vi "Event handler-Start Stop.vi"(9 "Next State":T1, 11 "UI queue":refnum<queue>) -> (0 "error out":errorcluster, 3 "Queue out":refnum<queue>)   [LabVIEW 2017]
uses:
  Queue/Message Queue/Typedefs/Message Cluster.ctl
  Typedefs/Top level VI states.ctl
  Typedefs/Set Main VI cursor.ctl
  Typedefs/Imaging Protocols enum.ctl
  Typedefs/Start-Stop Enum.ctl
  Global Variables/General Globals.vi
panel:
  # "<---Funct acq fix"
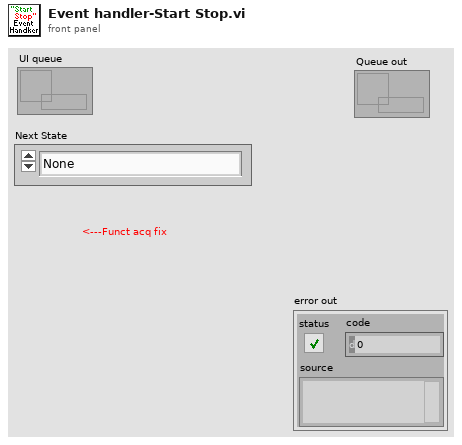
[diagram p1: front panel]
types:
  T1 = typedef "Top level VI states.ctl" = enum16{"None", "Initialise UI", "<STACK PROTOCOL STATES>", "AOL Zstack-START", "AOL Zstack-STOP", "Motor Zstack-START", "Motor Zstack-STOP", "<ACQUISITION PROTOCOL STATES> ", "Functional Acquisition-START", "Functional Acquisition-STOP", "Single Plane Acquisition-START", "Single Plane Acquisition-STOP", "Volume Acquisition-START", "Volume Acquisition-STOP", "<LIVE IMAGING PROTOCOL STATES>", "Live Imaging-START", "Live Imaging-STOP", "Live Plane Imaging-START", "Live Plane Imaging-STOP", "Live Volume Imaging-START", "Live Volume Imaging-STOP", "<MOVEMENT CORRECTION PROTOCOL STATES>", "EXIT"}
  T2 = typedef "Set Main VI cursor.ctl" = enum16{"Release busy cursor", "Set busy cursor"}
  T3 = typedef "Imaging Protocols enum.ctl" = enum16{"AOL Z-Stack", "Motor Z Stack", "Functional Acquisition", "Single Plane Acquisition", "Volume Acquisition", "Live Imaging", "Live Plane Imaging", "Live Volume Imaging"}
  T4 = typedef "Start-Stop Enum.ctl" = enum16{"START", "STOP"}
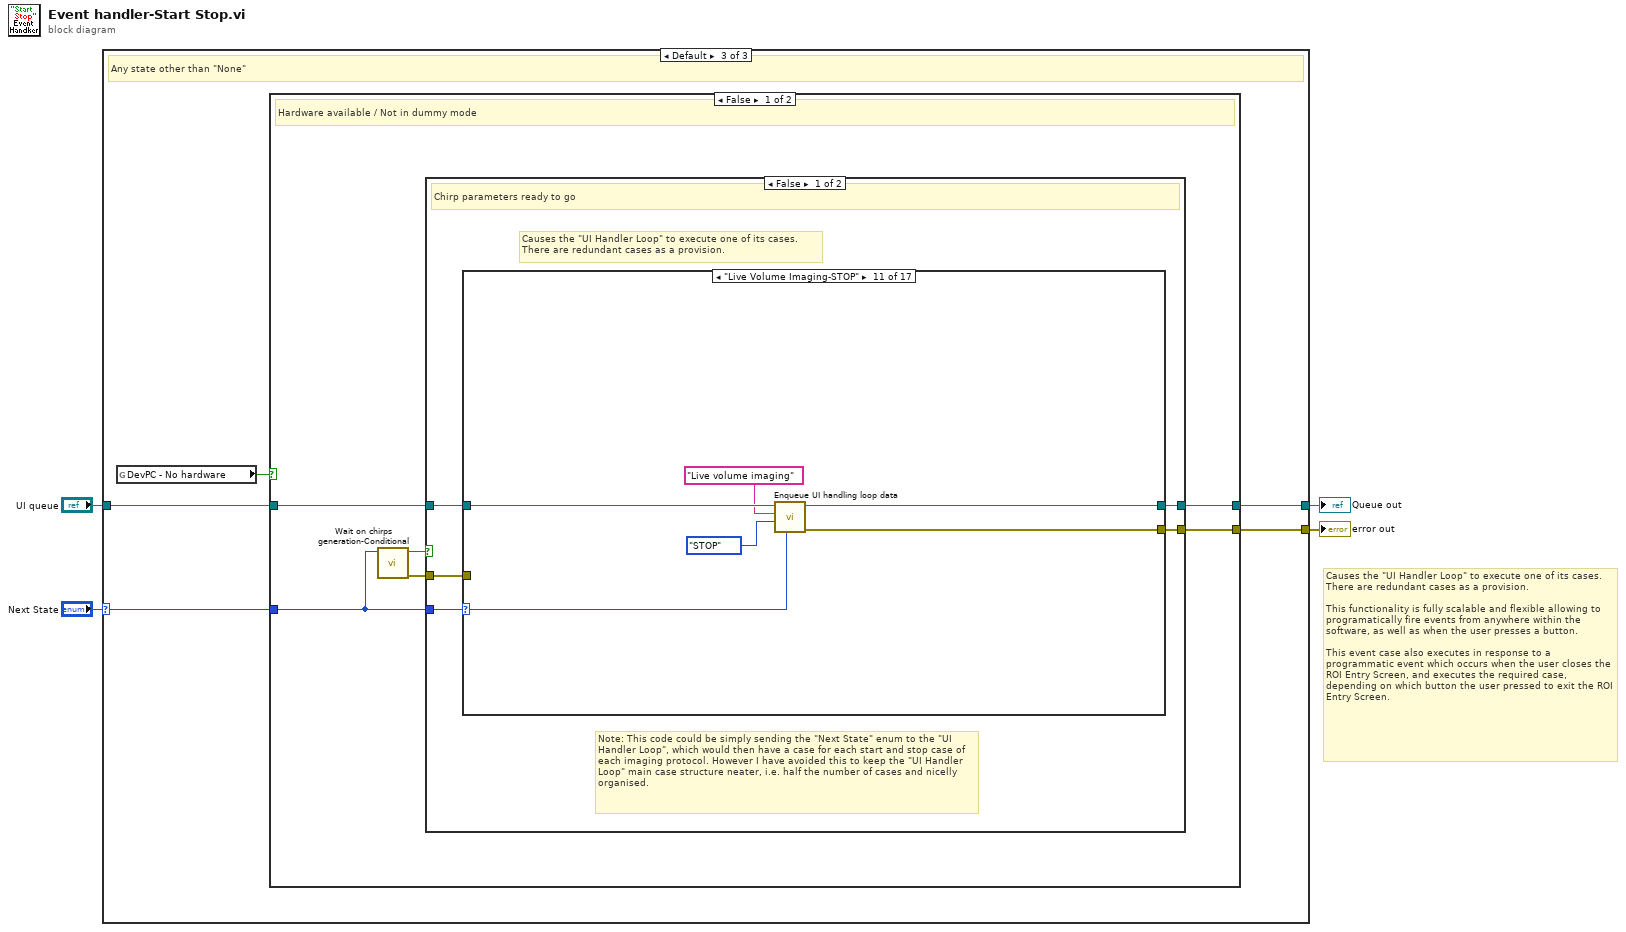
[diagram p0: block diagram]
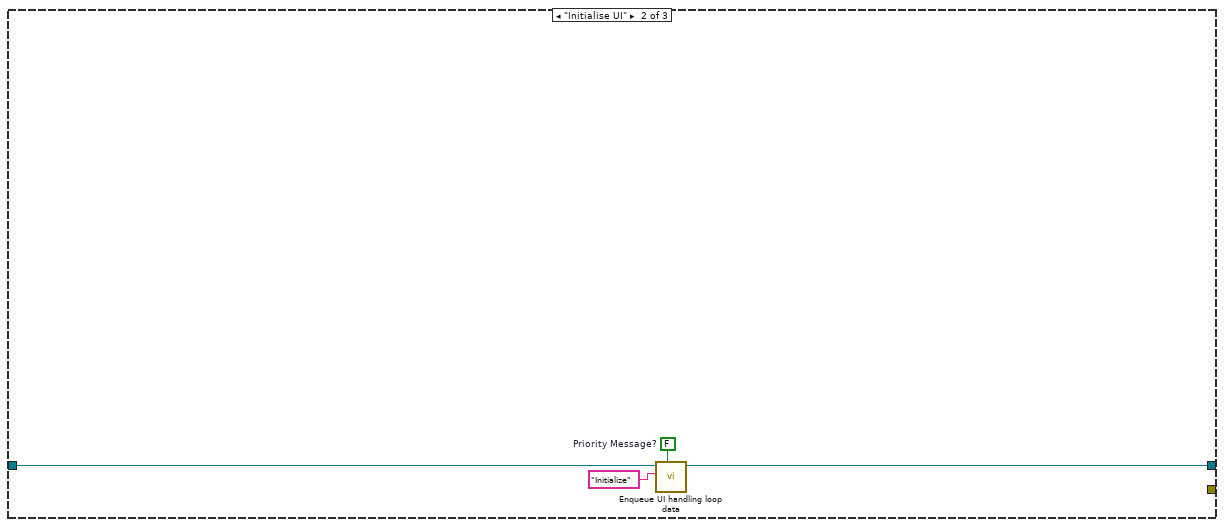
[diagram p3: hidden frame]
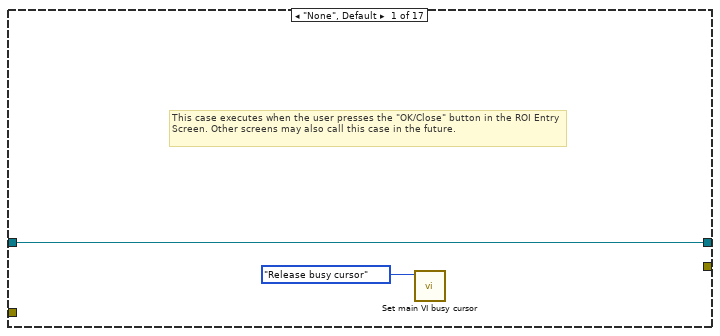
[diagram p4: hidden frame]
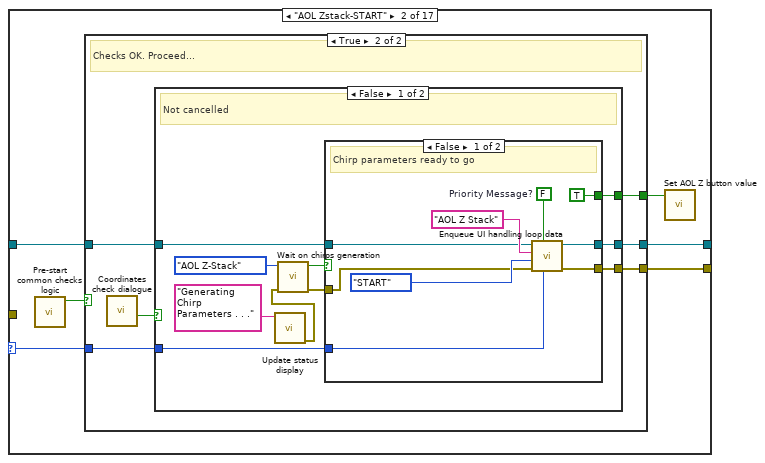
[diagram p5: hidden frame]
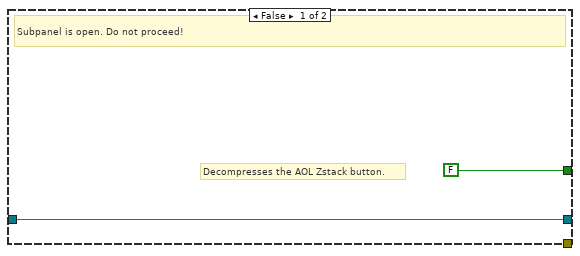
[diagram p6: hidden frame]
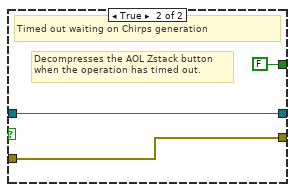
[diagram p7: hidden frame]
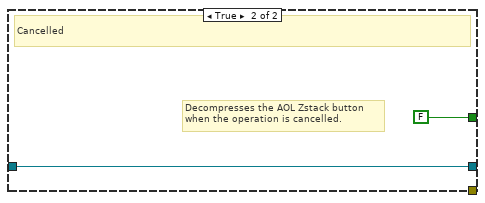
[diagram p8: hidden frame]
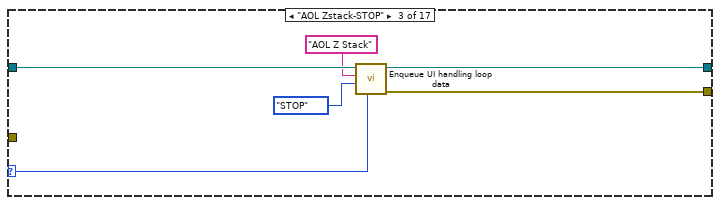
[diagram p9: hidden frame]
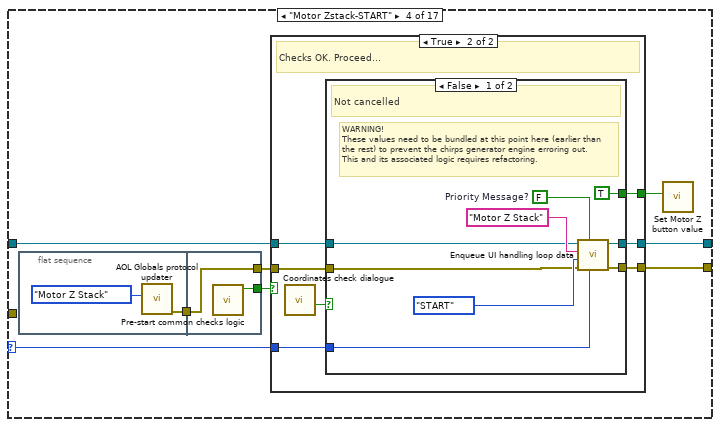
[diagram p10: hidden frame]
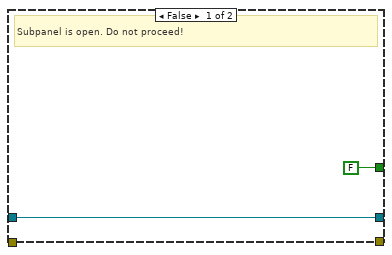
[diagram p11: hidden frame]
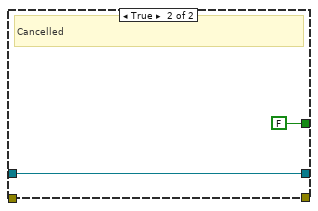
[diagram p12: hidden frame]
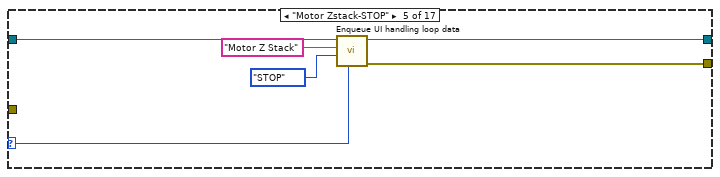
[diagram p13: hidden frame]
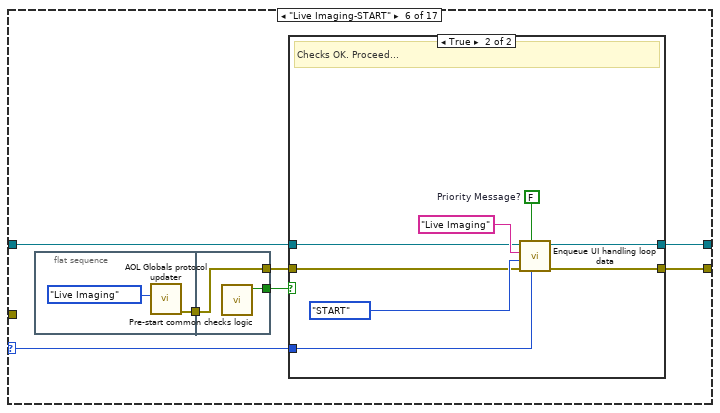
[diagram p14: hidden frame]
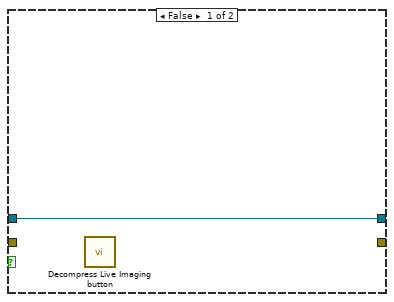
[diagram p15: hidden frame]
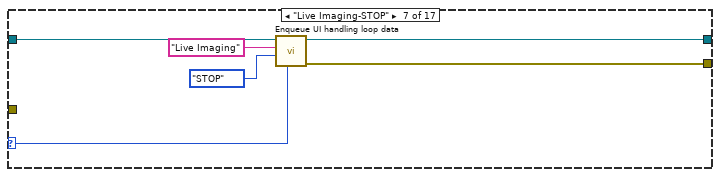
[diagram p16: hidden frame]
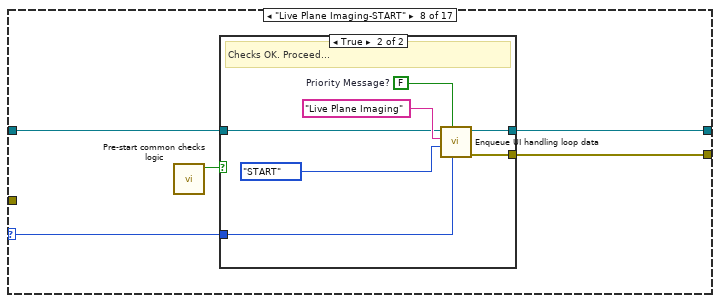
[diagram p17: hidden frame]
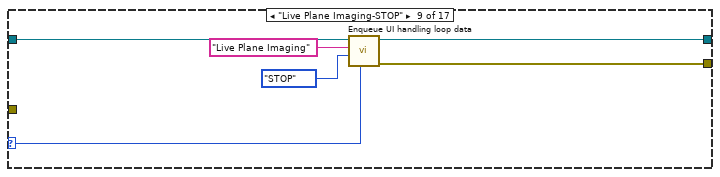
[diagram p19: hidden frame]
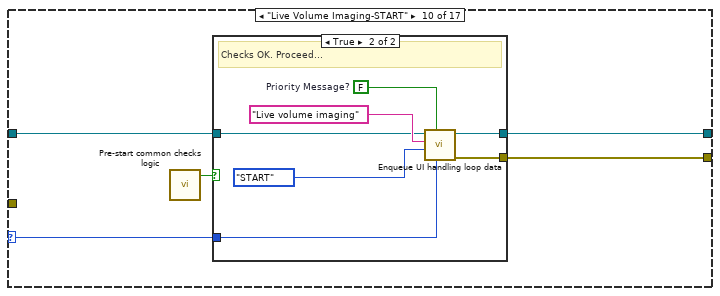
[diagram p20: hidden frame]
diagram:
  # "Causes the \"UI Handler Loop\" to execute one of its cases. There are redundant cases as a provision.\n\nThis functionality is fully scalable and flexible allowing to programatically fire events from anywhere within the software, as well as when the user presses a button.\n\nThis event case also executes in response to a programmatic event which occurs when the user closes the ROI Entry Screen, and executes the required case, depending on which button the user pressed to exit the ROI Entry Screen."
  n1 = case shown="Default" "Next State" {
    selector: "Next State" -> [_ _ w11]
    tunnel: "UI queue" -> [w5 w9 w14]
    tunnel: [_ _ w13] -> w3
    tunnel: [w5 w8 w12] -> w2
    frame "None" {
    }
    frame "Initialise UI" {
      w6 = FALSE  # Priority Message?
      n2 = call "Enqueue UI handling loop data.vi"("Priority Message? (T)"=w6, "Message"="Initialize", "Queue in"=w9) -> ("Queue out"=w8:refnum<queue>)  [unwired: 7 in, 1 out]
    }
    frame Default {
      # "Any state other than \"None\""
      n3 = global read "General Globals.vi" "DevPC - No hardware"() -> (w10:bool)
      n4 = case shown="False" w10 {
        tunnel: w14 -> [w20 w241]
        tunnel: [w19 _] -> w13
        tunnel: [w18 w241] -> w12
        tunnel: w11 -> [w17 w240]
        frame False {
          # "Hardware available / Not in dummy mode"
          n5 = call "Wait on chirps generation-Conditional.vi"("Next State"=w17) -> ("error out"=w15:errorcluster, "Timed out waiting on Chirps generation"=w16:bool)  [unwired: 9 in]
          n6 = case shown="False" w16 {
            tunnel: w20 -> [w25 w239]
            tunnel: w17 -> [w24 w236]
            tunnel: [w23 w237] -> w19
            tunnel: [w22 w239] -> w18
            tunnel: w15 -> [w21 w237]
            frame False {
              # "Note: This code could be simply sending the \"Next State\" enum to the \"UI Handler Loop\", which would then have a case for each start and stop case of each imaging protocol. However I have avoided this to keep the \"UI Handler Loop\" main case structure neater, i.e. half the number of cases and nicelly organised."
              # "Causes the \"UI Handler Loop\" to execute one of its cases.\nThere are redundant cases as a provision."
              # "Chirp parameters ready to go"
              n7 = case shown="\"Live Volume Imaging-STOP\"" w24 {
                selector: w24 -> [_ w29 w68 w77 w106 w115 w133 w139 w152 w158 w172 w177 w194 w200 w215 w219 w233]
                tunnel: w25 -> [w27 w33 w71 w79 w108 w113 w134 w138 w154 w156 w173 w179 w196 w202 w216 w221 w234]
                tunnel: [_ w32 w70 w78 w104 w116 w131 w140 w149 w159 w168 w178 w192 w201 w211 w220 w230] -> w23
                tunnel: [w27 w31 w67 w76 w105 w114 w132 w137 w150 w157 w169 w176 w193 w199 w212 w218 w231] -> w22
                tunnel: w21 -> [_ _ _ _ _ _ _ _ _ _ _ _ _ _ _ _ _]
                frame "None", Default {
                  # "This case executes when the user presses the \"OK/Close\" button in the ROI Entry Screen. Other screens may also call this case in the future."
                  n8 = call "Set main VI busy cursor.vi"("Main VI's cursor"=Set_Main_VI_cursor."Release busy cursor") -> ()  [unwired: 10 in, 1 out]
                }
                frame "AOL Zstack-START" {
                  n9 = call "Pre-start common checks logic.vi"() -> ("Proceed"=w30:bool)  [unwired: 11 in]
                  n10 = case shown="True" w30 {
                    tunnel: w33 -> [w35 w41]
                    tunnel: [_ w40] -> w32
                    tunnel: w29 -> [_ w39]
                    tunnel: [w35 w38] -> w31
                    tunnel: [FALSE ("Value") w36] -> w28
                    frame False {
                      # "Decompresses the AOL Zstack button."
                      # "Subpanel is open. Do not proceed!"
                    }
                    frame True {
                      # "Checks OK. Proceed..."
                      n11 = call "Coordinates check dialogue.vi"() -> ("Cancelled"=w37:bool)  [unwired: 11 in]
                      n12 = case shown="False" w37 {
                        tunnel: w41 -> [w46 w65]
                        tunnel: [w51 _] -> w40
                        tunnel: w39 -> [w49 _]
                        tunnel: [w50 w65] -> w38
                        tunnel: [w42 FALSE ("Value")] -> w36
                        frame False {
                          # "Not cancelled"
                          n13 = call "Update status display.vi"("Acquiring and Logging..."="Generating Chirp Parameters . . .") -> ("error out"=w44:errorcluster)  [unwired: 10 in]
                          n14 = call "Wait on chirps generation.vi"("error in (no error)"=w44, "Imaging Protocol"=Imaging_Protocols_enum."AOL Z-Stack") -> ("error out"=w43:errorcluster, "Timed out waiting on Chirps generation"=w47:bool)  [unwired: 8 in]
                          n15 = case shown="False" w47 {
                            tunnel: [w60 w62] -> w51
                            tunnel: w46 -> [w53 w63]
                            tunnel: [w58 w63] -> w50
                            tunnel: w49 -> [w55 _]
                            tunnel: w43 -> [w52 w62]
                            tunnel: [TRUE ("Value") FALSE ("Value")] -> w42
                            frame False {
                              w56 = FALSE  # Priority Message?
                              # "Chirp parameters ready to go"
                              n16 = call "Enqueue UI handling loop data.vi"("Next State"=w55, "Priority Message? (T)"=w56, "error in (no error)"=w52, "Start/Stop"=Start-Stop_Enum."START", "Message"="AOL Z Stack", "Queue in"=w53) -> ("error out"=w60:errorcluster, "Queue out"=w58:refnum<queue>)  [unwired: 4 in]
                            }
                            frame True {
                              # "Decompresses the AOL Zstack button\nwhen the operation has timed out."
                              # "Timed out waiting on Chirps generation"
                            }
                          }
                        }
                        frame True {
                          # "Decompresses the AOL Zstack button\nwhen the operation is cancelled."
                          # "Cancelled"
                        }
                      }
                    }
                  }
                  n17 = call "Set AOL Z button value.vi"("AOL Z button's new value"=w28) -> ()  [unwired: 10 in, 1 out]
                }
                frame "AOL Zstack-STOP" {
                  n18 = call "Enqueue UI handling loop data.vi"("Next State"=w68, "Start/Stop"=Start-Stop_Enum."STOP", "Message"="AOL Z Stack", "Queue in"=w71) -> ("error out"=w70:errorcluster, "Queue out"=w67:refnum<queue>)  [unwired: 6 in]
                }
                frame "Motor Zstack-START" {
                  n19 = flat-sequence {
                    tunnel: [w80] -> w75
                    tunnel: [w83] -> w74
                    tunnel: [w82] -> w73
                    tunnel: w75 -> [w82]
                    frame #0 {
                      n20 = call "AOL Globals protocol updater.vi"("Imaging Mode"=Imaging_Protocols_enum."Motor Z Stack") -> ("error out"=w80:errorcluster)  [unwired: 10 in]
                    }
                    frame #1 {
                      n21 = call "Pre-start common checks logic.vi"() -> ("Proceed"=w83:bool)  [unwired: 11 in]
                    }
                  }
                  n22 = case shown="True" w74 {
                    tunnel: w79 -> [w85 w92]
                    tunnel: [_ w91] -> w78
                    tunnel: w77 -> [_ w90]
                    tunnel: [w85 w89] -> w76
                    tunnel: w73 -> [_ w87]
                    tunnel: [FALSE w86] -> w72
                    frame False {
                      # "Subpanel is open. Do not proceed!"
                    }
                    frame True {
                      # "Checks OK. Proceed..."
                      n23 = call "Coordinates check dialogue.vi"() -> ("Cancelled"=w88:bool)  [unwired: 11 in]
                      n24 = case shown="False" w88 {
                        tunnel: w92 -> [w94 w103]
                        tunnel: [w100 _] -> w91
                        tunnel: w90 -> [w96 _]
                        tunnel: [w98 w103] -> w89
                        tunnel: w87 -> [w93 _]
                        tunnel: [TRUE FALSE] -> w86
                        frame False {
                          w97 = FALSE  # Priority Message?
                          # "WARNING!\nThese values need to be bundled at this point here (earlier than the rest) to prevent the chirps generator engine erroring out.\nThis and its associated logic requires refactoring."
                          # "Not cancelled"
                          n25 = call "Enqueue UI handling loop data.vi"("Next State"=w96, "Priority Message? (T)"=w97, "error in (no error)"=w93, "Start/Stop"=Start-Stop_Enum."START", "Message"="Motor Z Stack", "Queue in"=w94) -> ("error out"=w100:errorcluster, "Queue out"=w98:refnum<queue>)  [unwired: 4 in]
                        }
                        frame True {
                          # "Cancelled"
                        }
                      }
                    }
                  }
                  n26 = call "Set Motor Z button value.vi"("Motor Z button's new value"=w72) -> ()  [unwired: 10 in, 1 out]
                }
                frame "Motor Zstack-STOP" {
                  n27 = call "Enqueue UI handling loop data.vi"("Next State"=w106, "Start/Stop"=Start-Stop_Enum."STOP", "Message"="Motor Z Stack", "Queue in"=w108) -> ("error out"=w104:errorcluster, "Queue out"=w105:refnum<queue>)  [unwired: 6 in]
                }
                frame "Live Imaging-START" {
                  n28 = flat-sequence {
                    tunnel: [w117] -> w110
                    tunnel: [w120] -> w112
                    tunnel: [w119] -> w111
                    tunnel: w110 -> [w119]
                    frame #0 {
                      n29 = call "AOL Globals protocol updater.vi"("Imaging Mode"=Imaging_Protocols_enum."Live Imaging") -> ("error out"=w117:errorcluster)  [unwired: 10 in]
                    }
                    frame #1 {
                      n30 = call "Pre-start common checks logic.vi"() -> ("Proceed"=w120:bool)  [unwired: 11 in]
                    }
                  }
                  n31 = case shown="True" w112 {
                    tunnel: [_ w128] -> w116
                    tunnel: w115 -> [_ w124]
                    tunnel: [w121 w127] -> w114
                    tunnel: w113 -> [w121 w123]
                    tunnel: w111 -> [_ w122]
                    frame False {
                      n32 = call "Decompress Live Imaging button.vi"() -> ()  [unwired: 12 in]
                    }
                    frame True {
                      w125 = FALSE  # Priority Message?
                      # "Checks OK. Proceed..."
                      n33 = call "Enqueue UI handling loop data.vi"("Next State"=w124, "Priority Message? (T)"=w125, "error in (no error)"=w122, "Start/Stop"=Start-Stop_Enum."START", "Message"="Live Imaging", "Queue in"=w123) -> ("error out"=w128:errorcluster, "Queue out"=w127:refnum<queue>)  [unwired: 4 in]
                    }
                  }
                }
                frame "Live Imaging-STOP" {
                  n34 = call "Enqueue UI handling loop data.vi"("Next State"=w133, "Start/Stop"=Start-Stop_Enum."STOP", "Message"="Live Imaging", "Queue in"=w134) -> ("error out"=w131:errorcluster, "Queue out"=w132:refnum<queue>)  [unwired: 6 in]
                }
                frame "Live Plane Imaging-START" {
                  n35 = call "Pre-start common checks logic.vi"() -> ("Proceed"=w136:bool)  [unwired: 11 in]
                  n36 = case shown="True" w136 {
                    tunnel: [_ w148] -> w140
                    tunnel: w139 -> [_ w142]
                    tunnel: w138 -> [w141 w143]
                    tunnel: [w141 w146] -> w137
                    frame False {
                    }
                    frame True {
                      w145 = FALSE  # Priority Message?
                      # "Checks OK. Proceed..."
                      n37 = call "Enqueue UI handling loop data.vi"("Next State"=w142, "Priority Message? (T)"=w145, "Start/Stop"=Start-Stop_Enum."START", "Message"="Live Plane Imaging", "Queue in"=w143) -> ("error out"=w148:errorcluster, "Queue out"=w146:refnum<queue>)  [unwired: 5 in]
                    }
                  }
                }
                frame "Live Plane Imaging-STOP" {
                  n38 = call "Enqueue UI handling loop data.vi"("Next State"=w152, "Start/Stop"=Start-Stop_Enum."STOP", "Message"="Live Plane Imaging", "Queue in"=w154) -> ("error out"=w149:errorcluster, "Queue out"=w150:refnum<queue>)  [unwired: 6 in]
                }
                frame "Live Volume Imaging-START" {
                  n39 = call "Pre-start common checks logic.vi"() -> ("Proceed"=w155:bool)  [unwired: 11 in]
                  n40 = case shown="True" w155 {
                    tunnel: [_ w167] -> w159
                    tunnel: w158 -> [_ w162]
                    tunnel: [w160 w165] -> w157
                    tunnel: w156 -> [w160 w161]
                    frame False {
                    }
                    frame True {
                      w163 = FALSE  # Priority Message?
                      # "Checks OK. Proceed..."
                      n41 = call "Enqueue UI handling loop data.vi"("Next State"=w162, "Priority Message? (T)"=w163, "Start/Stop"=Start-Stop_Enum."START", "Message"="Live volume imaging", "Queue in"=w161) -> ("error out"=w167:errorcluster, "Queue out"=w165:refnum<queue>)  [unwired: 5 in]
                    }
                  }
                }
                frame "Live Volume Imaging-STOP" {
                  n42 = call "Enqueue UI handling loop data.vi"("Next State"=w172, "Start/Stop"=Start-Stop_Enum."STOP", "Message"="Live volume imaging", "Queue in"=w173) -> ("error out"=w168:errorcluster, "Queue out"=w169:refnum<queue>)  [unwired: 6 in]
                }
                frame "Functional Acquisition-START" {
                  n43 = call "Pre-start common checks logic.vi"() -> ("Proceed"=w174:bool)  [unwired: 11 in]
                  n44 = case shown="True" w174 {
                    tunnel: [FALSE ("Proceed") w181] -> w175
                    frame False {
                    }
                    frame True {
                      n45 = call "Funct acq pre-checks.vi"() -> ("Proceed"=w181:bool)  [unwired: 11 in]
                    }
                  }
                  n46 = case shown="True" w175 {
                    tunnel: w179 -> [w183 w184]
                    tunnel: [_ w191] -> w178
                    tunnel: w177 -> [_ w188]
                    tunnel: [w183 w189] -> w176
                    frame False {
                      # "Fail-safe logic.\nReleases the functional acquisition button if pressed."
                      # "Cannot be allowed to start"
                      n47 = call "Set Funct Acq button value.vi"("Functional Acquisition button's new value"=FALSE ("Value")) -> ()  [unwired: 10 in, 1 out]
                    }
                    frame True {
                      w186 = FALSE  # Priority Message?
                      w190 = Start-Stop_Enum."START"  # Main protocol
                      # "Allowed to start"
                      n48 = call "Set Funct Acq button value.vi"("Functional Acquisition button's new value"=TRUE ("Value")) -> ()  [unwired: 10 in, 1 out]
                      n49 = call "Enqueue UI handling loop data.vi"("Next State"=w188, "Priority Message? (T)"=w186, "Start/Stop"=w190, "Message"="Functional Acquisition", "Queue in"=w184) -> ("error out"=w191:errorcluster, "Queue out"=w189:refnum<queue>)  [unwired: 5 in]
                    }
                  }
                }
                frame "Functional Acquisition-STOP" {
                  # "Simply causes the UI to be re-enabled as soon as the functional data has been post processed (and displayed in the viewer where applicable)."
                  n50 = call "Enqueue UI handling loop data.vi"("Next State"=w194, "Start/Stop"=Start-Stop_Enum."STOP", "Message"="Functional Acquisition", "Queue in"=w196) -> ("error out"=w192:errorcluster, "Queue out"=w193:refnum<queue>)  [unwired: 6 in]
                }
                frame "Single Plane Acquisition-START" {
                  n51 = call "Pre-start common checks logic.vi"() -> ("Proceed"=w198:bool)  [unwired: 11 in]
                  n52 = case shown="True" w198 {
                    tunnel: w202 -> [w203 w204]
                    tunnel: [_ w210] -> w201
                    tunnel: w200 -> [_ w205]
                    tunnel: [w203 w209] -> w199
                    frame False {
                      # "ADD CODE HERE TO DECOMPRESS\nTHE FP BUTTON IF ONE IS ADDED LATER FOR THIS PROTOCOL."
                      # "May not start / HDD space low"
                    }
                    frame True {
                      w206 = FALSE  # Priority Message?
                      # "Allowed to start"
                      n53 = call "Enqueue UI handling loop data.vi"("Next State"=w205, "Priority Message? (T)"=w206, "Start/Stop"=Start-Stop_Enum."START", "Message"="Single Plane Acquisition", "Queue in"=w204) -> ("error out"=w210:errorcluster, "Queue out"=w209:refnum<queue>)  [unwired: 5 in]
                    }
                  }
                }
                frame "Single Plane Acquisition-STOP" {
                  n54 = call "Enqueue UI handling loop data.vi"("Next State"=w215, "Start/Stop"=Start-Stop_Enum."STOP", "Message"="Single Plane Acquisition", "Queue in"=w216) -> ("error out"=w211:errorcluster, "Queue out"=w212:refnum<queue>)  [unwired: 6 in]
                }
                frame "Volume Acquisition-START" {
                  n55 = call "Pre-start common checks logic.vi"() -> ("Proceed"=w217:bool)  [unwired: 11 in]
                  n56 = case shown="True" w217 {
                    tunnel: w221 -> [w222 w223]
                    tunnel: [_ w229] -> w220
                    tunnel: w219 -> [_ w224]
                    tunnel: [w222 w226] -> w218
                    frame False {
                      # "ADD CODE HERE TO DECOMPRESS\nTHE FP BUTTON IF ONE IS ADDED LATER FOR THIS PROTOCOL."
                      # "May not start / HDD space low"
                    }
                    frame True {
                      w225 = FALSE  # Priority Message?
                      # "Allowed to start"
                      n57 = call "Enqueue UI handling loop data.vi"("Next State"=w224, "Priority Message? (T)"=w225, "Start/Stop"=Start-Stop_Enum."START", "Message"="Volume acquisition", "Queue in"=w223) -> ("error out"=w229:errorcluster, "Queue out"=w226:refnum<queue>)  [unwired: 5 in]
                    }
                  }
                }
                frame "Volume Acquisition-STOP" {
                  n58 = call "Enqueue UI handling loop data.vi"("Next State"=w233, "Start/Stop"=Start-Stop_Enum."STOP", "Message"="Volume acquisition", "Queue in"=w234) -> ("error out"=w230:errorcluster, "Queue out"=w231:refnum<queue>)  [unwired: 6 in]
                }
              }
            }
            frame True {
              # "FAIL-SAFE CASE"
              # "Timed out waiting on Chirps generation"
              n59 = call "Stop case cleanup.vi"("Next State"=w236) -> ()  [unwired: 11 in]
              n60 = call "Set main VI busy cursor.vi"("Main VI's cursor"=Set_Main_VI_cursor."Release busy cursor") -> ()  [unwired: 10 in, 1 out]
            }
          }
        }
        frame True {
          # "Prevents execution start of all main functions when the hardware is unavailable (i.e. when dummy mode is active)"
          # "Dummy mode"
          n61 = flat-sequence {
            tunnel: w240 -> [w242]
            frame #0 {
              n62 = call "Set main VI busy cursor.vi"("Main VI's cursor"=Set_Main_VI_cursor."Release busy cursor") -> ()  [unwired: 10 in, 1 out]
              n63 = call "Stop case cleanup.vi"("Next State"=w242) -> ()  [unwired: 11 in]
            }
            frame #1 {
              n64 = call "Message Window.vi"("Message string"="This function cannot be used when the hardware is unavailable.") -> ()  [unwired: 10 in, 1 out]
            }
          }
        }
      }
    }
  }
  "error out" <- w3
  "Queue out" <- w2
